vi "Connect and publish.vi"() -> ()   [LabVIEW 2020, in "wamplv.lvlib"]
uses:
  wamplv.lvlib
  WAMP Client/WAMP Client.lvclass/WAMP Client.ctl
  WAMP Client/API/WAMP/Publish.vi/5e405bcd-0c6d-46be-a87b-06ec174a83c2.vi
  WAMP Client/API/WAMP/Publish (async).vi
  WAMP Client/Private/SubVIs/Raise Internal Message.vi
  WAMP Client/API/WAMP/Publish (async).vi/56cb05c7-ccfa-42e5-a428-2bd237dbc257.vi
  <vilib>/Utility/error.llb/Error Cluster From Error Code.vi
  WAMP Client/WAMP Client.lvclass
panel:
  in  "Arguments":string
  in  "Topic URI":string="test.topic"
  in  "Realm":string="default_realm"
  in  "Router URL":string="ws://localhost:8080/"
  # "Router URL examples: \n\ntcp://localhost:8080/ (RawSocket TCP)\ntcps://localhost:8080/ (RawSocket TCP with TLS/SSL)\nws://localhost:8080/ (WebScoket)\nws://localhost:8080/ws (WebScoket)\nwss://localhost:8080/ (WebSocket TCP with TLS/SSL)"
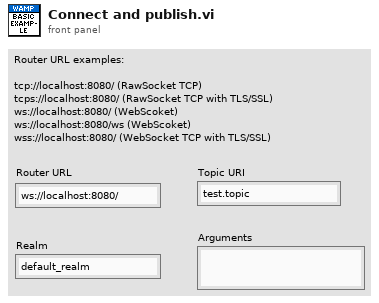
[diagram p1: front panel]
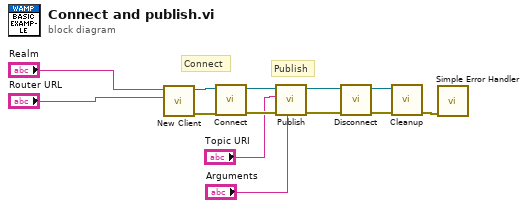
[diagram p0: block diagram]
diagram:
  # "Publish"
  # "Connect"
  n1 = call "New Client.vi"("Address"="Router URL", "Realm"="Realm") -> ("error out"=w8:errorcluster, "WAMP client out"=w11:refnum<class "WAMP Client.lvclass">)  [unwired: 8 in]
  n2 = call "Connect.vi"("error in"=w8, "WAMP Client in"=w11) -> ("error out"=w4:errorcluster, "WAMP Client out"=w6:refnum<class "WAMP Client.lvclass">)  [unwired: 8 in]
  n3 = call "Publish.vi"("Arguments"="Arguments", "Error in"=w4, "Topic"="Topic URI", "WAMP Client in"=w6) -> ("Error out"=w3:errorcluster, "WAMP Client out"=w5:refnum<class "WAMP Client.lvclass">)  [unwired: 5 in, 1 out]
  n4 = call-dynamic "Disconnect.vi"("error in"=w3, "WAMP Client in"=w5) -> ("error out"=w7:errorcluster, "WAMP Client out"=w10:refnum<class "WAMP Client.lvclass">)  [unwired: 8 in]
  n5 = call-dynamic "Cleanup.vi"("error in"=w7, "WAMP Client in"=w10) -> ("error out"=w9:errorcluster)  [unwired: 8 in, 1 out]
  n6 = call <vilib>:"Simple Error Handler.vi"("error in (no error)"=w9) -> ()  [unwired: 4 in, 5 out]
